vi "filter sampled data.vi"(7 "low cutoff freq: fl":dbl=30.0 format="%0.4f", 10 "t x data":cluster{"t":dbl[], "x":dbl[]}) -> (2 "t x data filetered":cluster{"t":dbl[], "x":dbl[]})   [LabVIEW 2010]
uses:
  <vilib>/Analysis/3filter.llb/Filter Passband Type.ctl
  <vilib>/Analysis/3filter.llb/Bessel Filter (DBL).vi
  <vilib>/gmath/NI_Gmath.lvlib
  <vilib>/Analysis/NI_AALBase.lvlib
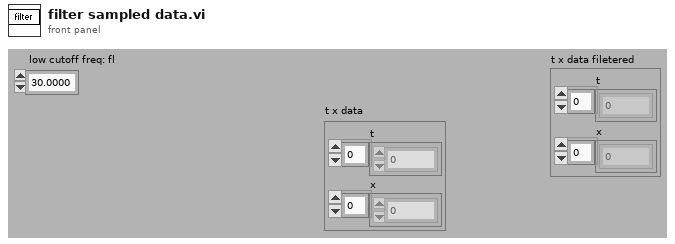
[diagram p1: front panel]
types:
  T1 = typedef "NI_AALBase.lvlib/Filter Passband Type.ctl" = enum32{"Lowpass", "Highpass", "Bandpass", "Bandstop"}
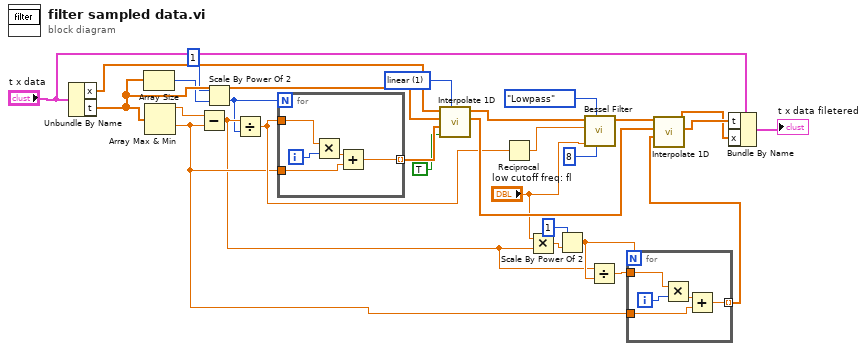
[diagram p0: block diagram]
diagram:
  w23 = 1 items=["nearest", "linear", "spline", "cubic Hermite", "Lagrange"] ("method")
  n1 = Unbundle By Name("t x data") -> ("x"=w27:dbl[], "t"=w26:dbl[])
  n2 = Array Size(array=w26) -> (size(s)=w2:i32)
  n3 = Array Max & Min(array=w26) -> (max value=w28:dbl, min value=w12:dbl)  [unwired: 2 out]
  n4 = Subtract(x=w28, y=w12) -> (x-y=w9:dbl)
  n5 = Scale By Power Of 2(n=1, x=w2) -> (x*2^n=w3:i32)
  n6 = Divide(x=w9, y=w3) -> (x/y=w16:dbl)
  n7 = for {
    N: w3 -> [_]
    tunnel: w16 -> [w32]
    tunnel: w12 -> [w30]
    tunnel: [w29] -> w25 mode=indexing
    i -> [w33]
    n8 = Multiply(x=w32, y=w33) -> (x*y=w31:dbl)
    n9 = Add(x=w31, y=w30) -> (x+y=w29:dbl)
  }
  n10 = call <vilib>:"Interpolate 1D.vi"("method"=w23, "X is monotonic"=TRUE, "xi"=w25, "X"=w26, "Y"=w27) -> ("xi used"=w17:dbl[], "yi"=w20:dbl[])  [unwired: 4 in, 1 out]
  n11 = Reciprocal(x=w16) -> (1/x=w19:dbl)
  n12 = Multiply(x="low cutoff freq: fl", y=w9) -> (x*y=w14:dbl)
  n13 = Scale By Power Of 2(n=1, x=w14) -> (x*2^n=w10:dbl)
  n14 = call-poly <vilib>:"Bessel Filter.vi"("order"=8, "filter type"=Filter_Passband_Type."Lowpass", "low cutoff freq: fl"="low cutoff freq: fl", "sampling freq: fs"=w19, "X"=w20) -> ("Filtered X"=w18:dbl[])  [unwired: 3 in, 1 out]
  n15 = Divide(x=w9, y=w10) -> (x/y=w11:dbl)
  n16 = for {
    N: w10 -> [_]
    tunnel: w11 -> [w37]
    tunnel: w12 -> [w35]
    tunnel: [w34] -> w8 mode=indexing
    i -> [w38]
    n17 = Multiply(x=w37, y=w38) -> (x*y=w36:dbl)
    n18 = Add(x=w36, y=w35) -> (x+y=w34:dbl)
  }
  n19 = call <vilib>:"Interpolate 1D.vi"("xi"=w8, "X"=w17, "Y"=w18) -> ("xi used"=w7:dbl[], "yi"=w6:dbl[])  [unwired: 6 in, 1 out]
  n20 = Bundle By Name(cluster="t x data", "t"=w7, "x"=w6) -> (→"t x data filetered":cluster{"t":dbl[], "x":dbl[]})
